vi "Test Circular Buffer.vi"() -> ()   [LabVIEW 2015, in "Circular Buffer.lvclass"]
uses:
  Circular Buffer.lvclass
panel:
  out "Values 2":dbl[](array[numeric])
  out "error out":errorcluster
  out "Values":dbl[](array[numeric])
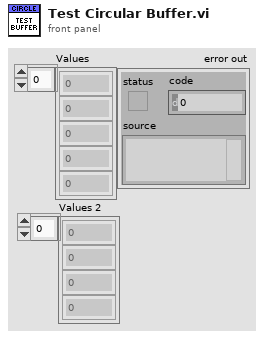
[diagram p1: front panel]
types:
  T1 = typedef "Circular Buffer.lvclass/Session Handle.ctl" = refnum<data-value>
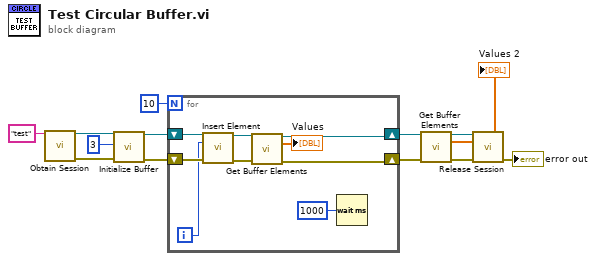
[diagram p0: block diagram]
diagram:
  n1 = call "Obtain Session.vi"("Session  Name ()"="test") -> ("Session Handle"=w12:T1, "error out"=w11:errorcluster)  [unwired: 13 in]
  n2 = call "Initialize Buffer.vi"("Session Handle in"=w12, "Size"=u16 3, "error in (no error)"=w11) -> ("Session Handle out"=w8:T1, "error out"=w7:errorcluster)  [unwired: 11 in]
  n3 = for {
    N: 10 -> [_]
    shift-right: [w16] -> w6
    shift-left: w8 -> [w22]
    shift-right: [w17] -> w5
    shift-left: w7 -> [w21]
    i -> [w20]
    n4 = call "Insert Element.vi"("Session Handle in"=w22, "Value"=w20, "error in (no error)"=w21) -> ("Session Handle out"=w19:T1, "error out"=w18:errorcluster)  [unwired: 11 in]
    n5 = call "Get Buffer Elements.vi"("Session Handle in"=w19, "error in (no error)"=w18) -> ("Session Handle out"=w16:T1, "Values"=→"Values":dbl[], "error out"=w17:errorcluster)  [unwired: 10 in, 1 out]
    n6 = Wait (ms)(milliseconds to wait=u32 1000) -> ()  [unwired: 1 out]
  }
  n7 = call "Get Buffer Elements.vi"("Session Handle in"=w6, "error in (no error)"=w5) -> ("Session Handle out"=w4:T1, "Values"=→"Values 2":dbl[], "error out"=w3:errorcluster)  [unwired: 10 in, 1 out]
  n8 = call "Release Session.vi"("Session Handle"=w4, "error in (no error)"=w3) -> ("error out"=→"error out":errorcluster)  [unwired: 13 in]
